vi "SMO.Dictionary.TestLauncher.vi"() -> ()   [LabVIEW 2013, in "SMO.Dictionary.lvlib" / "SMO.Dictionary.lvclass"]
uses:
  SMO.Dictionary.lvclass
  <vilib>/JKI/JKI SMO/SMO/Typedefs/SMOState --Enum.ctl
  <vilib>/JKI/JKI SMO/SMO/SMO.lvclass/SMO.ctl
  <vilib>/JKI/JKI SMO/SMO/Private/ReftoDVR--SMO.vi
  <vilib>/JKI/JKI SMO/SMO/SMO.lvclass
panel:
  out "SMO State":T1
  out "error out":errorcluster
  in  "Stop":bool
  # "Dictionary Test Launcher"
  # "For instructions on how to use the JKI State Machine Objects, examples and video tutorials, visit:\nhttp://jki.net/state-machine-objects/\n\nJKI State Machine Objects™\nhttp://jki.net/state-machine-objects/\nCopyright (C) 2005-2015, JKI <info@jki.net>\nALL RIGHTS RESERVED"
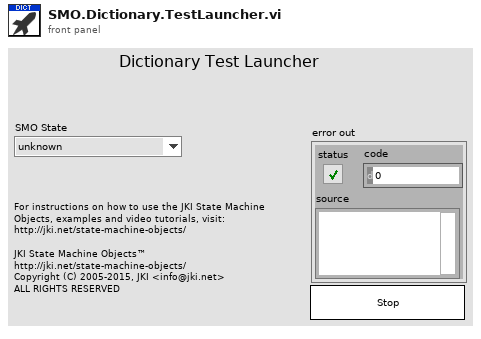
[diagram p1: front panel]
types:
  T1 = typedef "SMO.lvclass/SMOState --Enum.ctl" = enum16{"unknown", "Created", "Started", "Stopped"}
  T2 = typedef "SMO.lvclass/Public Events.ctl" = cluster{"Error":refnum<user-event>, "State":refnum<user-event>, "Reserve State":refnum<user-event>}
  T3 = cluster{"Event Registration Refnum":refnum<event-registration>}
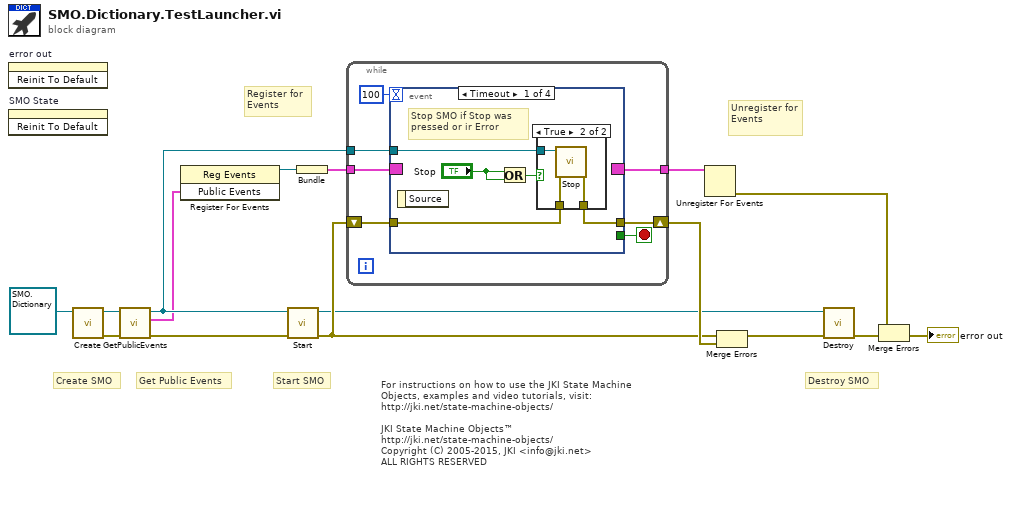
[diagram p0: block diagram]
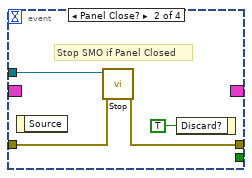
[diagram p3: hidden frame]
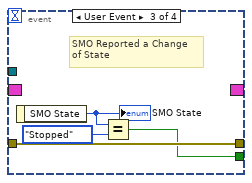
[diagram p4: hidden frame]
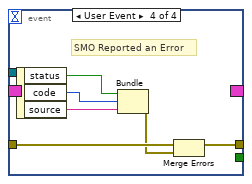
[diagram p5: hidden frame]
diagram:
  # "For instructions on how to use the JKI State Machine Objects, examples and video tutorials, visit:\nhttp://jki.net/state-machine-objects/\n\nJKI State Machine Objects™\nhttp://jki.net/state-machine-objects/\nCopyright (C) 2005-2015, JKI <info@jki.net>\nALL RIGHTS RESERVED"
  # "Get Public Events"
  # "Start SMO"
  # "Destroy SMO"
  # "Create SMO"
  # "Unregister for Events"
  # "Register for Events"
  n1 = invoke on="error out" class="Clust (strict)" method="Reinit To Default"() -> ()  [unwired: 3 in, 3 out]
  n2 = invoke on="SMO State" class="Enum (strict)" method="Reinit To Default"() -> ()  [unwired: 3 in, 3 out]
  n3 = call <vilib>:"Create.vi"("SMO"=refnum<class "SMO.Dictionary.lvclass"> refnum ("SMO.Template.lvclass")) -> ("error out"=w5:errorcluster, "SMO out"=w6:refnum<class "SMO.Dictionary.lvclass">)  [unwired: 8 in, 1 out]
  n4 = call <vilib>:"GetPublicEvents.vi"("error in (no error)"=w5, "SMO"=w6) -> ("error out"=w4:errorcluster, "Public Events"=w2:T2, "SMO out"=w3:refnum<class "SMO.Dictionary.lvclass">)  [unwired: 7 in]
  n5 = register-events(w2) -> (reference out=w1:refnum<event-registration>)  [unwired: 2 in, 1 out]
  n6 = call <vilib>:"Start.vi"("error in (no error)"=w4, "SMO"=w3) -> ("error out"=w9:errorcluster, "SMO out"=w7:refnum<class "SMO.Dictionary.lvclass">)  [unwired: 8 in]
  n7 = Bundle("Event Registration Refnum"=w1) -> (w15:T3)  [unwired: 1 in]
  n8 = while {
    shift-right: [w22] -> w14
    shift-left: w9 -> [w21]
    tunnel: w15 -> [w20]
    tunnel: [w19] -> w16
    tunnel: w3 -> [w18]
    stop <- w23 stop-if-true
    n9 = event shown="[0] Timeout" {
      selector: w20 -> [_ _ _ _]
      dyn-events: [_ _ _ _] -> w19
      timeout: 100 -> [_ _ _ _]
      tunnel: [_ _ w37 _] -> w23
      tunnel: w18 -> [w28 w36 _ _]
      tunnel: [w27 w35 w40 w44] -> w22
      tunnel: w21 -> [w26 w34 w40 w42]
      event Timeout {
        # "Stop SMO if Stop was \npressed or ir Error"
        n10 = event-data() -> ()  [unwired: 1 in, 1 out]
        n11 = Or(x="Stop", y="Stop") -> (x .or. y?=w25:bool)
        n12 = case shown="True" w25 {
          tunnel: w28 -> [_ w32]
          tunnel: [w29 w31] -> w27
          tunnel: w26 -> [w29 w30]
          frame False {
          }
          frame True {
            n13 = call <vilib>:"Stop.vi"("error in (no error)"=w30, "SMO"=w32) -> ("error out"=w31:errorcluster)  [unwired: 8 in, 1 out]
          }
        }
      }
      event Panel Close? {
        # "Stop SMO if Panel Closed"
        n14 = event-data() -> ()  [unwired: 1 in, 1 out]
        n15 = call <vilib>:"Stop.vi"("error in (no error)"=w34, "SMO"=w36) -> ("error out"=w35:errorcluster)  [unwired: 8 in, 1 out]
        n16 = event-data("Discard?"=TRUE ("OK")) -> ()  [unwired: 1 in, 1 out]
      }
      event User Event {
        # "SMO Reported a Change\nof State"
        n17 = event-data() -> ("SMO State"=w39:T1)  [unwired: 1 in]
        "SMO State" <- w39
        n18 = Equal?(x=w39, y=SMOState_--Enum."Stopped") -> (x = y?=w37:bool)
      }
      event User Event {
        # "SMO Reported an Error"
        n19 = event-data() -> ("status"=w43:bool, "code"=w46:i32, "source"=w45:string)  [unwired: 1 in]
        n20 = Bundle("status"=w43, "code"=w46, "source"=w45) -> (w41:errorcluster)  [unwired: 1 in]
        n21 = Merge Errors(w42, w41) -> (w44:errorcluster)
      }
    }
  }
  n22 = Unregister For Events(event registration refnum=w16) -> (error out=w13:errorcluster)  [unwired: 1 in]
  n23 = Merge Errors(w9, w14) -> (w8:errorcluster)
  n24 = call <vilib>:"Destroy.vi"("error in (no error)"=w8, "SMO"=w7) -> ("error out"=w11:errorcluster)  [unwired: 9 in]
  n25 = Merge Errors(w13, w11) -> (→"error out":errorcluster)
